vi "PathPlanner_PathFinder_ComputeOrImprovePath.vi"(8 "error in (no error)":errorcluster) -> (0 "error out":errorcluster)   [LabVIEW 2019]
uses:
  PathPlannerLib24/VI/PathPlanner_GridPosition_FromHash.vi
  PathPlannerLib24/VI/PathPlanner_PathFinder_Heuristic.vi
  PathPlannerLib24/VI/PathPlanner_GridPosition_Get.vi
  PathPlannerLib24/VI/PathPlanner_PathFinder_Cost.vi
  PathPlannerLib24/VI/PathPlanner_GridPosition_Equals.vi
  PathPlannerLib24/VI/PathPlanner_GridPosition_New.vi
  PathPlannerLib24/VI/PathPlanner_PathFinder_IsCollision.vi
  PathPlannerLib24/VI/PathPlanner_GridPosition_Print.vi
  PathPlannerLib24/VI/PathPlanner_PathFinder_Globals.vi
  PathPlannerLib24/PathPlanner24.lvlib
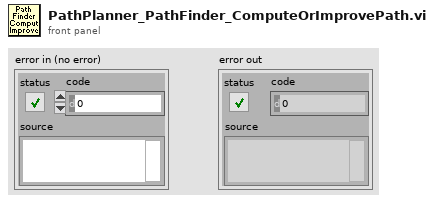
[diagram p1: front panel]
types:
  T1 = typedef "PathPlanner24.lvlib/PathPlannerFinderDoublePair.ctl" = cluster{"A":dbl, "B":dbl}
  T2 = typedef "PathPlanner24.lvlib/PathPlannerFinderGridPosition.ctl" = cluster{"X":i32, "Y":i32}
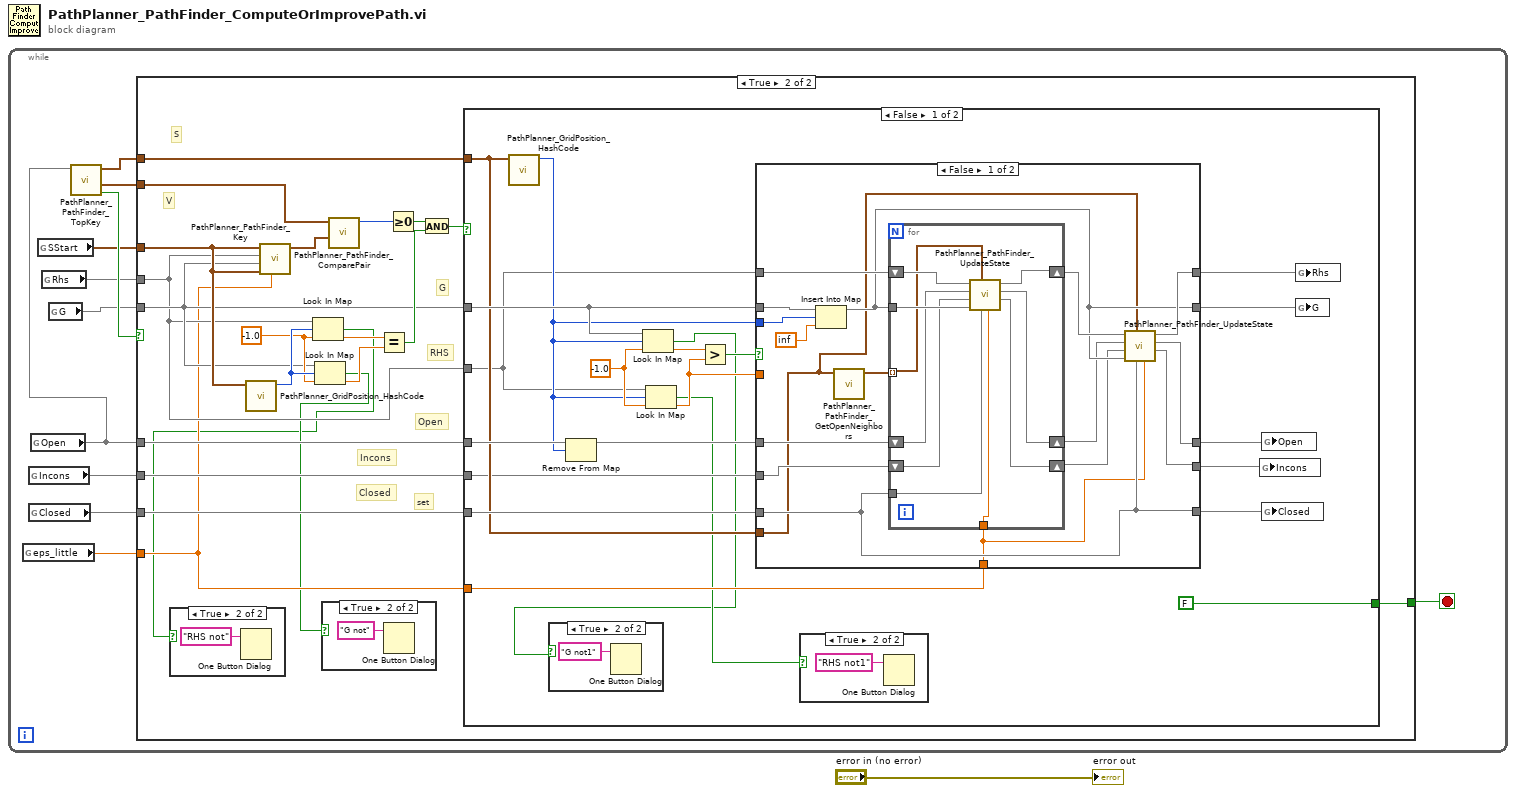
[diagram p0: block diagram]
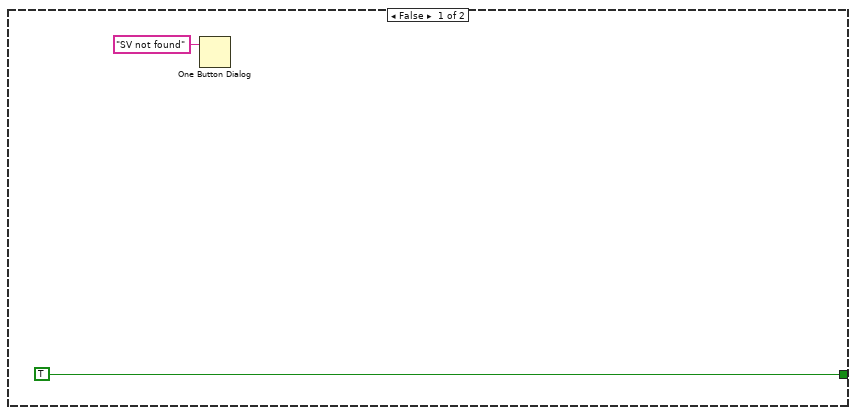
[diagram p2: hidden frame]
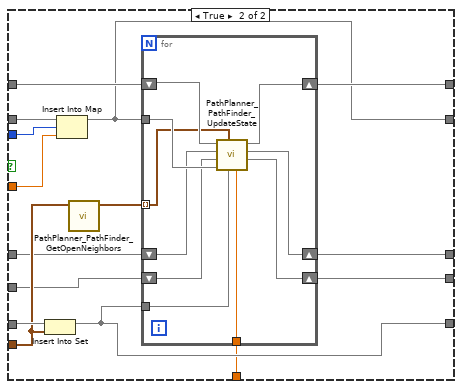
[diagram p7: hidden frame]
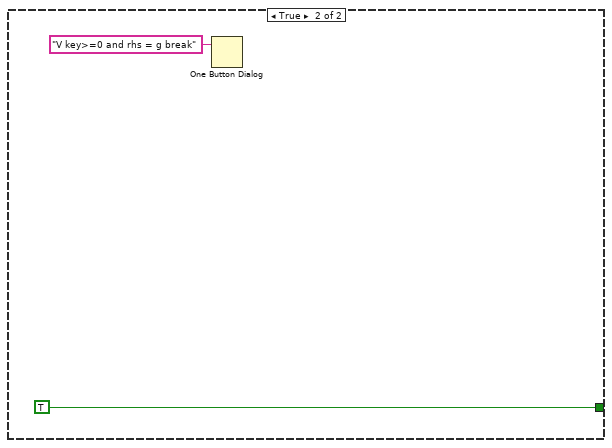
[diagram p8: hidden frame]
diagram:
  n1 = while {
    stop <- w11 stop-if-true
    n2 = global read "PathPlanner_PathFinder_Globals.vi" "eps_little"() -> (w2:dbl)
    n3 = global read "PathPlanner_PathFinder_Globals.vi" "Incons"() -> (w4:map{i32, T1})
    n4 = global read "PathPlanner_PathFinder_Globals.vi" "Closed"() -> (w5:set{T2})
    n5 = global read "PathPlanner_PathFinder_Globals.vi" "Open"() -> (w3:map{i32, T1})
    n6 = global read "PathPlanner_PathFinder_Globals.vi" "SStart"() -> (w8:T2)
    n7 = global read "PathPlanner_PathFinder_Globals.vi" "Rhs"() -> (w7:map{i32, dbl})
    n8 = global read "PathPlanner_PathFinder_Globals.vi" "G"() -> (w6:map{i32, dbl})
    n9 = call "PathPlanner_PathFinder_TopKey.vi"("Open"=w3) -> ("Found"=w12:bool, "DoublePair"=w9:T1, "PathPlannerFinderGridPosition"=w10:T2)  [unwired: 8 in]
    n10 = case shown="True" w12 {
      tunnel: [TRUE w24] -> w11
      tunnel: w10 -> [_ w22]
      tunnel: w9 -> [_ w35]
      tunnel: w8 -> [_ w31]
      tunnel: w7 -> [_ w20]
      tunnel: w6 -> [_ w21]
      tunnel: w3 -> [_ w23]
      tunnel: w5 -> [_ w19]
      tunnel: w4 -> [_ w18]
      tunnel: w2 -> [_ w17]
      frame False {
        n11 = One Button Dialog(message="SV not found") -> ()  [unwired: 1 in, 1 out]
      }
      frame True {
        w29 = -1.0 ("default value")
        # "Incons"
        # "set"
        # "Closed"
        # "RHS"
        # "Open"
        # "G"
        # "S"
        # "V"
        n12 = call "PathPlanner_GridPosition_HashCode.vi"("GridPosition"=w31) -> ("HashCode"=w30:i32)  [unwired: 10 in]
        n13 = call "PathPlanner_PathFinder_Key.vi"("eps_little"=w17, "Sstart"=w31, "G"=w21, "RHS"=w20, "S"=w31) -> ("DoublePair"=w34:T1)  [unwired: 6 in]
        n14 = Look In Map(map=w20, key=w30, default value=w29) -> (key not found?=w15:bool, value=w28:dbl)
        n15 = case shown="True" w15 {
          frame False {
          }
          frame True {
            n16 = One Button Dialog(message="RHS not") -> ()  [unwired: 1 in, 1 out]
          }
        }
        n17 = Look In Map(map=w21, key=w30, default value=w29) -> (key not found?=w16:bool, value=w27:dbl)
        n18 = case shown="True" w16 {
          frame False {
          }
          frame True {
            n19 = One Button Dialog(message="G not") -> ()  [unwired: 1 in, 1 out]
          }
        }
        n20 = call "PathPlanner_PathFinder_ComparePair.vi"("B"=w34, "A"=w35) -> ("Compare"=w33:i32)  [unwired: 9 in]
        n21 = Equal?(x=w28, y=w27) -> (x = y?=w26:bool)
        n22 = Greater Or Equal To 0?(x=w33) -> (x >= 0?=w32:bool)
        n23 = And(x=w32, y=w26) -> (x .and. y?=w25:bool)
        n24 = case shown="False" w25 {
          tunnel: [FALSE TRUE] -> w24
          tunnel: w23 -> [w58 _]
          tunnel: w22 -> [w50 _]
          tunnel: w21 -> [w54 _]
          tunnel: w20 -> [w49 _]
          tunnel: w19 -> [w51 _]
          tunnel: w18 -> [w47 _]
          tunnel: w17 -> [w40 _]
          frame False {
            w57 = -1.0 ("default value")
            n25 = call "PathPlanner_GridPosition_HashCode.vi"("GridPosition"=w50) -> ("HashCode"=w53:i32)  [unwired: 10 in]
            n26 = Remove From Map(10:w53, 11:w58) -> (3:w48:map{i32, T1})  [unwired: 2 out]
            n27 = Look In Map(map=w54, key=w53, default value=w57) -> (key not found?=w38:bool, value=w56:dbl)
            n28 = case shown="True" w38 {
              frame False {
              }
              frame True {
                n29 = One Button Dialog(message="G not1") -> ()  [unwired: 1 in, 1 out]
              }
            }
            n30 = Look In Map(map=w49, key=w53, default value=w57) -> (key not found?=w39:bool, value=w52:dbl)
            n31 = Greater?(x=w56, y=w52) -> (0:w55:bool)
            n32 = case shown="False" w55 {
              tunnel: w54 -> [w77 w102]
              tunnel: w53 -> [w76 w101]
              tunnel: w52 -> [_ w100]
              tunnel: w51 -> [w63 w99]
              tunnel: w50 -> [w62 w98]
              tunnel: [w63 w90] -> w46
              tunnel: [w68 w89] -> w42
              tunnel: w49 -> [w74 w96]
              tunnel: [w69 w95] -> w43
              tunnel: w48 -> [w72 w94]
              tunnel: [w66 w93] -> w44
              tunnel: w47 -> [w71 w92]
              tunnel: [w64 w91] -> w45
              tunnel: w40 -> [w61 w88]
              frame False {
                n33 = Insert Into Map(map in=w77, key=w76, value=inf) -> (map out=w68:map{i32, dbl})  [unwired: 2 out]
                n34 = call "PathPlanner_PathFinder_GetOpenNeighbors.vi"("GridPosition S"=w62) -> ("Open Neighbors"=w73:T2[])  [unwired: 10 in]
                n35 = for {
                  shift-right: [w86] -> w70
                  shift-left: w74 -> [w87]
                  shift-right: [w83] -> w67
                  shift-left: w72 -> [w84]
                  shift-right: [w81] -> w65
                  shift-left: w71 -> [w82]
                  tunnel: w73 -> [w79] mode=indexing
                  tunnel: w68 -> [w85]
                  tunnel: w63 -> [w80]
                  tunnel: w61 -> [w78]
                  n36 = call "PathPlanner_PathFinder_UpdateState.vi"("eps_Little"=w78, "Closed"=w80, "S"=w79, "G"=w85, "Incons"=w82, "Open"=w84, "RHS"=w87) -> ("Incons out"=w81:map{i32, T1}, "Open out"=w83:map{i32, T1}, "RHS out"=w86:map{i32, dbl})  [unwired: 2 in]
                }
                n37 = call "PathPlanner_PathFinder_UpdateState.vi"("eps_Little"=w61, "Closed"=w63, "S"=w62, "G"=w68, "Incons"=w65, "Open"=w67, "RHS"=w70) -> ("Incons out"=w64:map{i32, T1}, "Open out"=w66:map{i32, T1}, "RHS out"=w69:map{i32, dbl})  [unwired: 2 in]
              }
              frame True {
                n38 = Insert Into Set(10:w98, 11:w99) -> (3:w90:set{T2})  [unwired: 1 out]
                n39 = Insert Into Map(map in=w102, key=w101, value=w100) -> (map out=w89:map{i32, dbl})  [unwired: 2 out]
                n40 = call "PathPlanner_PathFinder_GetOpenNeighbors.vi"("GridPosition S"=w98) -> ("Open Neighbors"=w97:T2[])  [unwired: 10 in]
                n41 = for {
                  tunnel: w97 -> [w105] mode=indexing
                  shift-right: [w111] -> w95
                  shift-left: w96 -> [w112]
                  shift-right: [w108] -> w93
                  shift-left: w94 -> [w109]
                  shift-right: [w106] -> w91
                  shift-left: w92 -> [w107]
                  tunnel: w89 -> [w110]
                  tunnel: w90 -> [w104]
                  tunnel: w88 -> [w103]
                  n42 = call "PathPlanner_PathFinder_UpdateState.vi"("eps_Little"=w103, "Closed"=w104, "S"=w105, "G"=w110, "Incons"=w107, "Open"=w109, "RHS"=w112) -> ("Incons out"=w106:map{i32, T1}, "Open out"=w108:map{i32, T1}, "RHS out"=w111:map{i32, dbl})  [unwired: 2 in]
                }
              }
            }
            n43 = case shown="True" w39 {
              frame False {
              }
              frame True {
                n44 = One Button Dialog(message="RHS not1") -> ()  [unwired: 1 in, 1 out]
              }
            }
            n45 = global write "PathPlanner_PathFinder_Globals.vi" "Incons"(w45) -> ()
            n46 = global write "PathPlanner_PathFinder_Globals.vi" "Open"(w44) -> ()
            n47 = global write "PathPlanner_PathFinder_Globals.vi" "Closed"(w46) -> ()
            n48 = global write "PathPlanner_PathFinder_Globals.vi" "Rhs"(w43) -> ()
            n49 = global write "PathPlanner_PathFinder_Globals.vi" "G"(w42) -> ()
          }
          frame True {
            n50 = One Button Dialog(message="V key>=0 and rhs = g break") -> ()  [unwired: 1 in, 1 out]
          }
        }
      }
    }
  }
  "error out" <- "error in (no error)"
